vi "Load Freq List.vi"(8 "error in (no error)":errorcluster, 11 "Freq List file":path=path "D:/Valeo/Micriphone Test/Config/ME79_NewFreqcsv") -> (0 "error out":errorcluster, 1 "Freq for THD":cluster{"Numeric":dbl, "Numeric":dbl}[](array[cluster]), 2 "Frequency List":T1(array[cluster]), 3 "Spec List":cluster{"Lower":dbl, "Upper":dbl}[](array[cluster]), 5 "appended array":cluster{dbl[], dbl[]}[](array[cluster]))   [LabVIEW 2018]
uses:
  <vilib>/Utility/file.llb/Read Delimited Spreadsheet (DBL).vi
panel:
  out "XY Graph":cluster{dbl[], dbl[]}[](graph)
  out "output cluster":cluster{dbl[], dbl[], dbl[]}
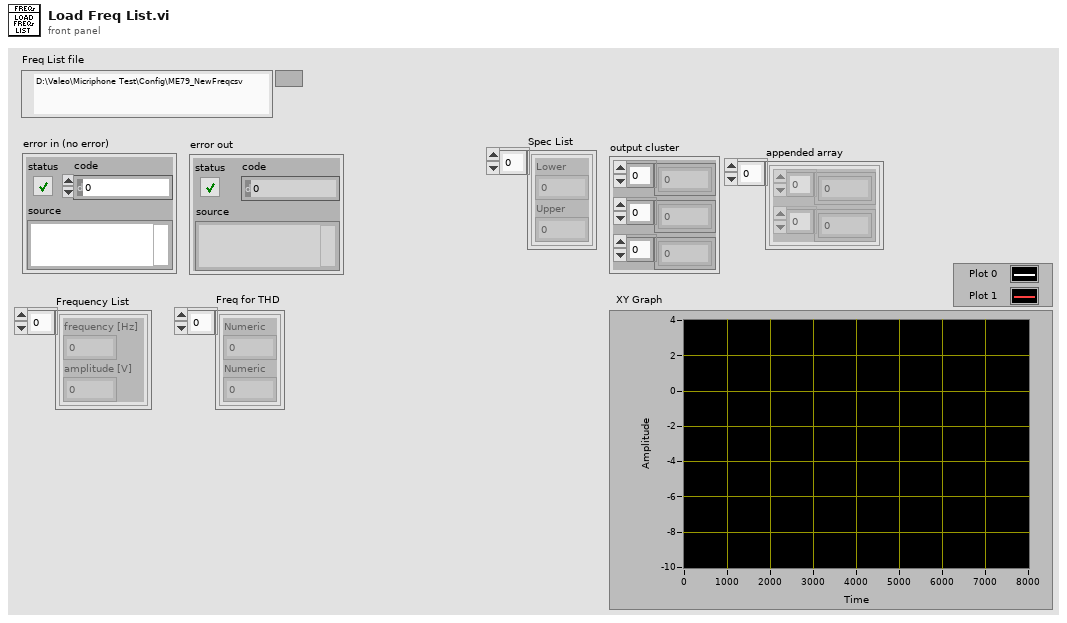
[diagram p1: front panel]
types:
  T1 = cluster{"frequency [Hz]":dbl, "amplitude [V]":dbl}[]
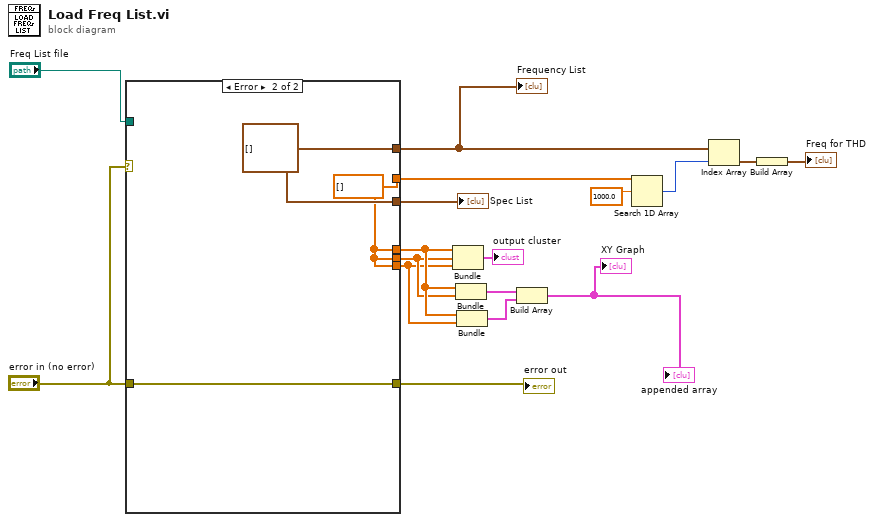
[diagram p0: block diagram]
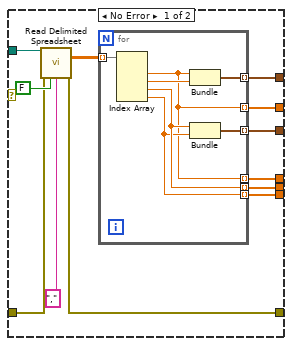
[diagram p2: hidden frame]
diagram:
  n1 = case shown="Error" "error in (no error)" {
    tunnel: "Freq List file" -> [w29 _]
    tunnel: [w25 w39] -> w16
    tunnel: "error in (no error)" -> [w26 w39]
    tunnel: [w23 w38] -> w11
    tunnel: [w22 w37] -> w12
    tunnel: [w21 w38] -> w8
    tunnel: [w20 w37] -> w5
    tunnel: [w19 w37] -> w2
    tunnel: [w18 w37] -> w6
    frame No Error {
      n2 = call-poly <vilib>:"Read Delimited Spreadsheet.vi"("file path (dialog if empty)"=w29, "error in (no error)"=w26, "transpose? (F)"=FALSE, "delimiter (\\t)"="," ("delimiter (\\t)")) -> ("all rows"=w24:dbl[][], "error out"=w25:errorcluster)  [unwired: 6 in, 4 out]
      n3 = for {
        tunnel: w24 -> [w36] mode=indexing
        tunnel: [w34] -> w23 mode=indexing
        tunnel: [w30] -> w22 mode=indexing
        tunnel: [w33] -> w21 mode=indexing
        tunnel: [w32] -> w20 mode=indexing
        tunnel: [w31] -> w19 mode=indexing
        tunnel: [w30] -> w18 mode=indexing
        n4 = Index Array(array=w36) -> (element #1=w30:dbl, element #2=w35:dbl, element #3=w32:dbl, element #4=w31:dbl)  [unwired: 4 in]
        n5 = Bundle("Numeric"=w30, "Numeric"=w35) -> (w34:cluster{"Numeric":dbl, "Numeric":dbl})  [unwired: 1 in]
        n6 = Bundle("Numeric"=w32, "Numeric"=w31) -> (w33:cluster{"Numeric":dbl, "Numeric":dbl})  [unwired: 1 in]
      }
    }
    frame Error {
      w37 = dbl[] []
      w38 = cluster{"Numeric":dbl, "Numeric":dbl}[] []
    }
  }
  "error out" <- w16
  "Frequency List" <- w11
  "Spec List" <- w8
  n7 = Bundle(w6, w5, w2) -> (→"output cluster":cluster{dbl[], dbl[], dbl[]})  [unwired: 1 in]
  n8 = Bundle(w6, w5) -> (w4:cluster{dbl[], dbl[]})  [unwired: 1 in]
  n9 = Bundle(w6, w2) -> (w1:cluster{dbl[], dbl[]})  [unwired: 1 in]
  n10 = Build Array(w4, w1) -> (→"XY Graph" →"appended array":cluster{dbl[], dbl[]}[])
  n11 = Search 1D Array(1D array=w12, element=1000.0 ("index")) -> (index of element=w13:i32)  [unwired: 1 in]
  n12 = Index Array(array=w11, index=w13) -> (element=w10:cluster{"Numeric":dbl, "Numeric":dbl})
  n13 = Build Array(w10) -> (→"Freq for THD":cluster{"Numeric":dbl, "Numeric":dbl}[])
